vi "[subVI]_parse_distance_data_and_CRC.vi"(11 "S300 data (input)":string) -> (3 "distance data and CRC":string, 4 "Stop?":bool)   [LabVIEW 2013]
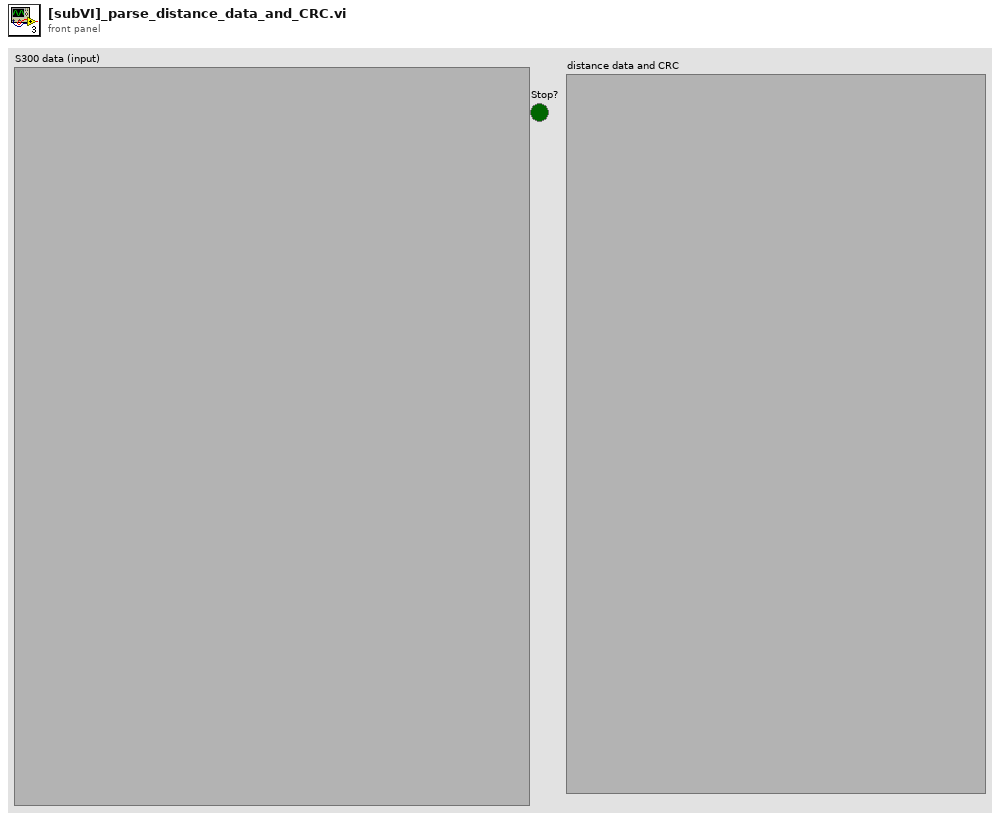
[diagram p1: front panel]
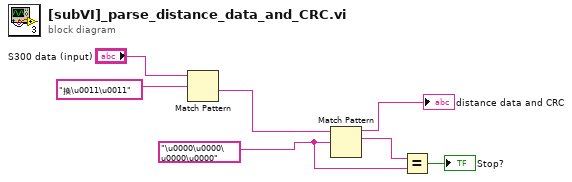
[diagram p0: block diagram]
diagram:
  w1 = "\u0000\u0000\u0000\u0000"
  n1 = Match Pattern(string="S300 data (input)", regular expression="换\u0011\u0011") -> (after substring=w5:string)  [unwired: 1 in, 3 out]
  n2 = Match Pattern(string=w5, regular expression=w1) -> (before substring=→"distance data and CRC":string, match substring=w4:string)  [unwired: 1 in, 2 out]
  n3 = Equal?(x=w4, y=w1) -> (x = y?=→"Stop?":bool)
